vi "init.vi"(8 "error in":errorcluster, 10 "TBM module configuration in":refnum<class "TBM module configuration.lvclass">, 11 "fixed channel runtime in":refnum<class "DAQmx Watchdog runtime.lvclass">) -> (0 "error out":errorcluster, 1 "data allocations":T1, 2 "execution settings":T4, 3 "fixed channel runtime out":refnum<class "DAQmx Watchdog runtime.lvclass">)   [LabVIEW 2014, in "DAQmx Watchdog runtime.lvclass"]
doc: "Provides an interface for initializing a module at runtime. While this interface performs no operations, a child should provide an override which may open any necessary references or sessions, allocate necessary memory, and perform any final configuration validataion before providing the full configuration <b>execution data</b> to the calling process."
uses:
  DAQmx Watchdog runtime.lvclass
  <vilib>/NI/Tag Bus Module Framework/module configuration/TBM module configuration.lvclass
  <vilib>/NI/Tag Bus Module Framework/runtime/execution settings.ctl
  <vilib>/NI/Tag Bus Module Framework/channel/data tables.ctl
  <vilib>/NI/Tag Bus/dictionary/data dictionary.lvclass
  <vilib>/NI/Tag Bus/dictionary table pair.ctl
  <vilib>/NI/Tag Bus/table/data table.ctl
  configuration/DAQmx Watchdog configuration.lvclass
  DAQmx Watchdog runtime.lvclass/DAQmx Watchdog runtime.ctl
  <vilib>/DAQmx/configure/task.llb/DAQmx Configure Watchdog Expiration States (Analog Output).vi
  <vilib>/DAQmx/configure/task.llb/DAQmx Configure Watchdog Expiration States (Counter Output).vi
  <vilib>/DAQmx/configure/task.llb/DAQmx Configure Watchdog Expiration States (Digital Output).vi
  <vilib>/NI/DCAF/Tag Editor Core/control module/runtime/control module runtime.lvclass
  <resource>/objmgr/daqmx.rc
  <vilib>/NI/Tag Bus Module Framework/runtime/TBM module execution interface.lvclass
  <vilib>/NI/Tag Bus Module Framework/channel/TBM channel.lvclass
  <vilib>/NI/Tag Bus/tag bus.lvlib
  <vilib>/NI/Tag Bus/table/data table.lvlib
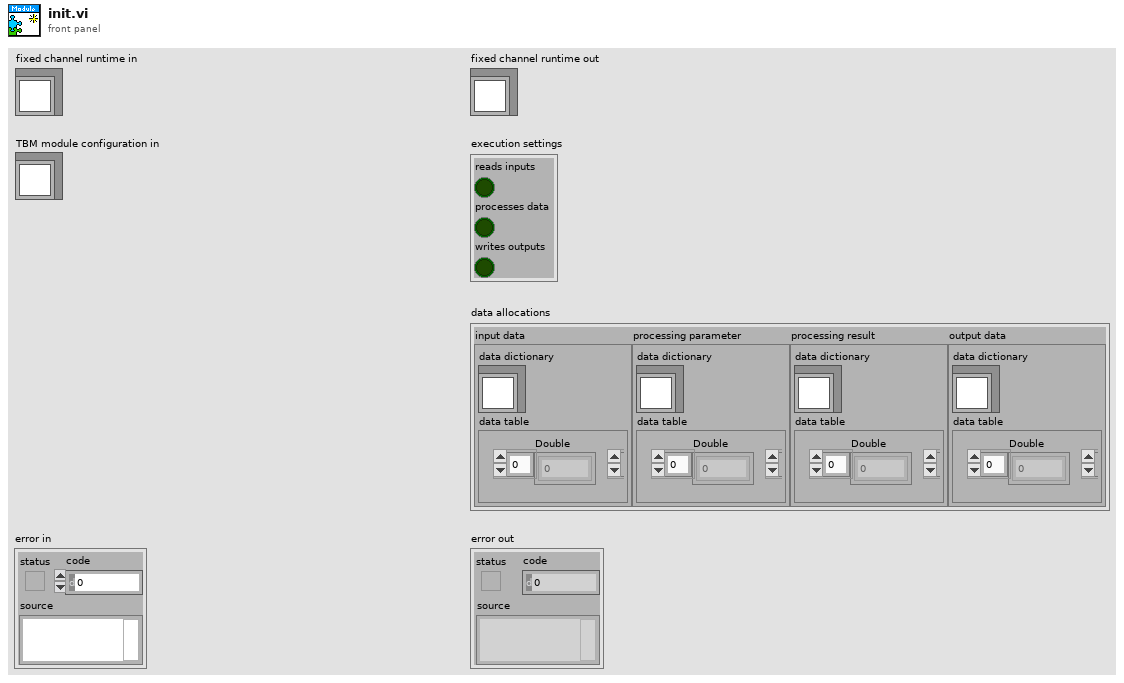
[diagram p1: front panel]
types:
  T1 = typedef "TBM channel.lvclass/data tables.ctl" = cluster{"input data":T2, "processing parameter":T2, "processing result":T2, "output data":T2}
  T2 = typedef "tag bus.lvlib/dictionary table pair.ctl" = cluster{"data dictionary":refnum<class "data dictionary.lvclass">, "data table":T3}
  T3 = typedef "tag bus.lvlib/data table.lvlib/data table.ctl" = cluster{"Double":dbl[], "Single":sgl[], "I64":i64[], "I32":i32[], "I16":i16[], "I8":i8[], "U64":u64[], "U32":u32[], "U16":u16[], "U8":u8[], "Boolean":bool[], "String":string[], "Array of Double":cluster{"DBL Array":dbl[]}[], "Array of Single":cluster{"SGL Array":sgl[]}[], "Array of I64":cluster{"I64 Array":i64[]}[], "Array of I32":cluster{"I32 Array":i32[]}[], "Array of I16":cluster{"I16 Array":i16[]}[], "Array of I8":cluster{"I8 Array":i8[]}[], "Array of U64":cluster{"U64 Array":u64[]}[], "Array of U32":cluster{"U32 Array":u32[]}[], "Array of U16":cluster{"U16 Array":u16[]}[], "Array of U8":cluster{"U8 Array":u8[]}[], "Array of Boolean":cluster{"Boolean Array":bool[]}[], "Array of String":cluster{"String Array":string[]}[]}
  T4 = typedef "TBM module execution interface.lvclass/execution settings.ctl" = cluster{"reads inputs":bool, "processes data":bool, "writes outputs":bool}
  T5 = cluster{"physical channel":tag, "expiration state":dbl, "output type":i32}[]
  T6 = cluster{"physical channel(s)":tag, "expiration state":i32}[]
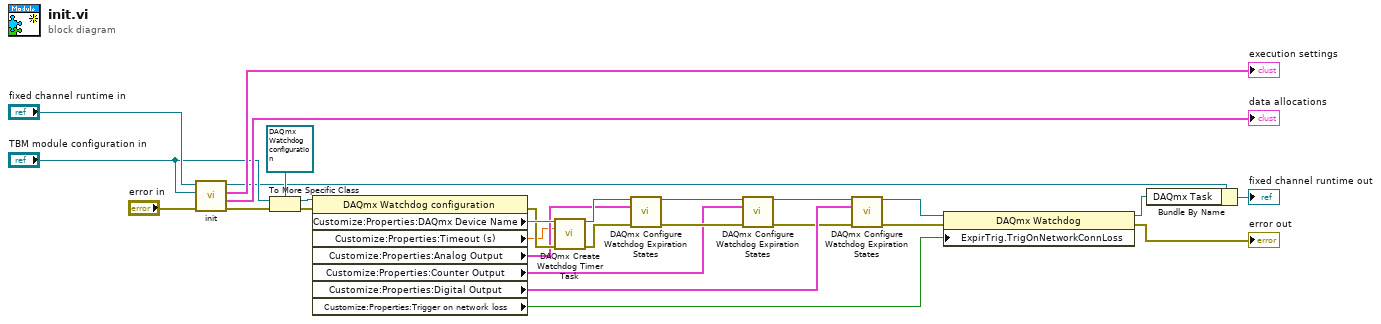
[diagram p0: block diagram]
diagram:
  n1 = call-parent "init.vi"("error in"="error in", "TBM module configuration in"="TBM module configuration in", "fixed channel runtime in"="fixed channel runtime in") -> ("error out"=w19:errorcluster, "data allocations"=→"data allocations":T1, "execution settings"=→"execution settings":T4, "fixed channel runtime out"=w4:refnum<class "DAQmx Watchdog runtime.lvclass">)  [unwired: 5 in]
  n2 = To More Specific Class(target class=refnum<class "DAQmx Watchdog configuration.lvclass"> refnum, reference="TBM module configuration in", error in=w19) -> (specific class reference=w22:refnum<class "DAQmx Watchdog configuration.lvclass">, error out=w23:errorcluster)
  n3 = property class="DAQmx Watchdog configuration"(reference=w22, error in=w23) -> (error out=w20:errorcluster, "Customize:Properties:DAQmx Device Name"=w21:tag, "Customize:Properties:Timeout (s)"=w12:dbl, "Customize:Properties:Analog Output"=w16:T5, "Customize:Properties:Counter Output"=w13:T6, "Customize:Properties:Digital Output"=w10:T6, "Customize:Properties:Trigger on network loss"=w6:bool)  [unwired: 1 out]
  n4 = call <vilib>:"DAQmx Create Watchdog Timer Task.vi"("device in"=w21, "timeout"=w12, "error in"=w20) -> ("task out"=w18:refnum<k21>, "error out"=w17:errorcluster)  [unwired: 11 in]
  n5 = call-poly <vilib>:"DAQmx Configure Watchdog Expiration States.vi"("task in"=w18, "expiration states"=w16, "error in"=w17) -> ("task out"=w14:refnum<k21>, "error out"=w15:errorcluster)  [unwired: 11 in]
  n6 = call-poly <vilib>:"DAQmx Configure Watchdog Expiration States.vi"("task in"=w14, "expiration states"=w13, "error in"=w15) -> ("task out"=w11:refnum<k21>, "error out"=w9:errorcluster)  [unwired: 11 in]
  n7 = call-poly <vilib>:"DAQmx Configure Watchdog Expiration States.vi"("task in"=w11, "expiration states"=w10, "error in"=w9) -> ("task out"=w8:refnum<k21>, "error out"=w7:errorcluster)  [unwired: 11 in]
  n8 = property class="DAQmx Watchdog"(reference=w8, error in=w7, "ExpirTrig.TrigOnNetworkConnLoss"=w6) -> (reference out=w2:refnum<k21>, error out=→"error out":errorcluster)
  n9 = Bundle By Name(cluster=w4, "DAQmx Task"=w2) -> (→"fixed channel runtime out":refnum<class "DAQmx Watchdog runtime.lvclass">)
